vi "VI Tree.vi"   [LabVIEW 2020, in "Rohde&Schwarz CMWXP NR FR1 Measurement.lvlib"]
doc: "This is the instrument driver for the Rohde&Schwarz CMWXP NR FR1 Measurement. \n\nThe VI Tree displays all the user-callable VIs of the instrument driver in an organized table.\n\nFor detailed driver information including modification history, refer to the <B>rscmwxpnrfr1m.chm </B>file."
uses:
  <instrlib>/Rohde&Schwarz CMWXP NR FR1 Measurement/Rohde&Schwarz CMWXP NR FR1 Measurement.lvlib
panel:
  # "rsCmwxpNrFr1M"
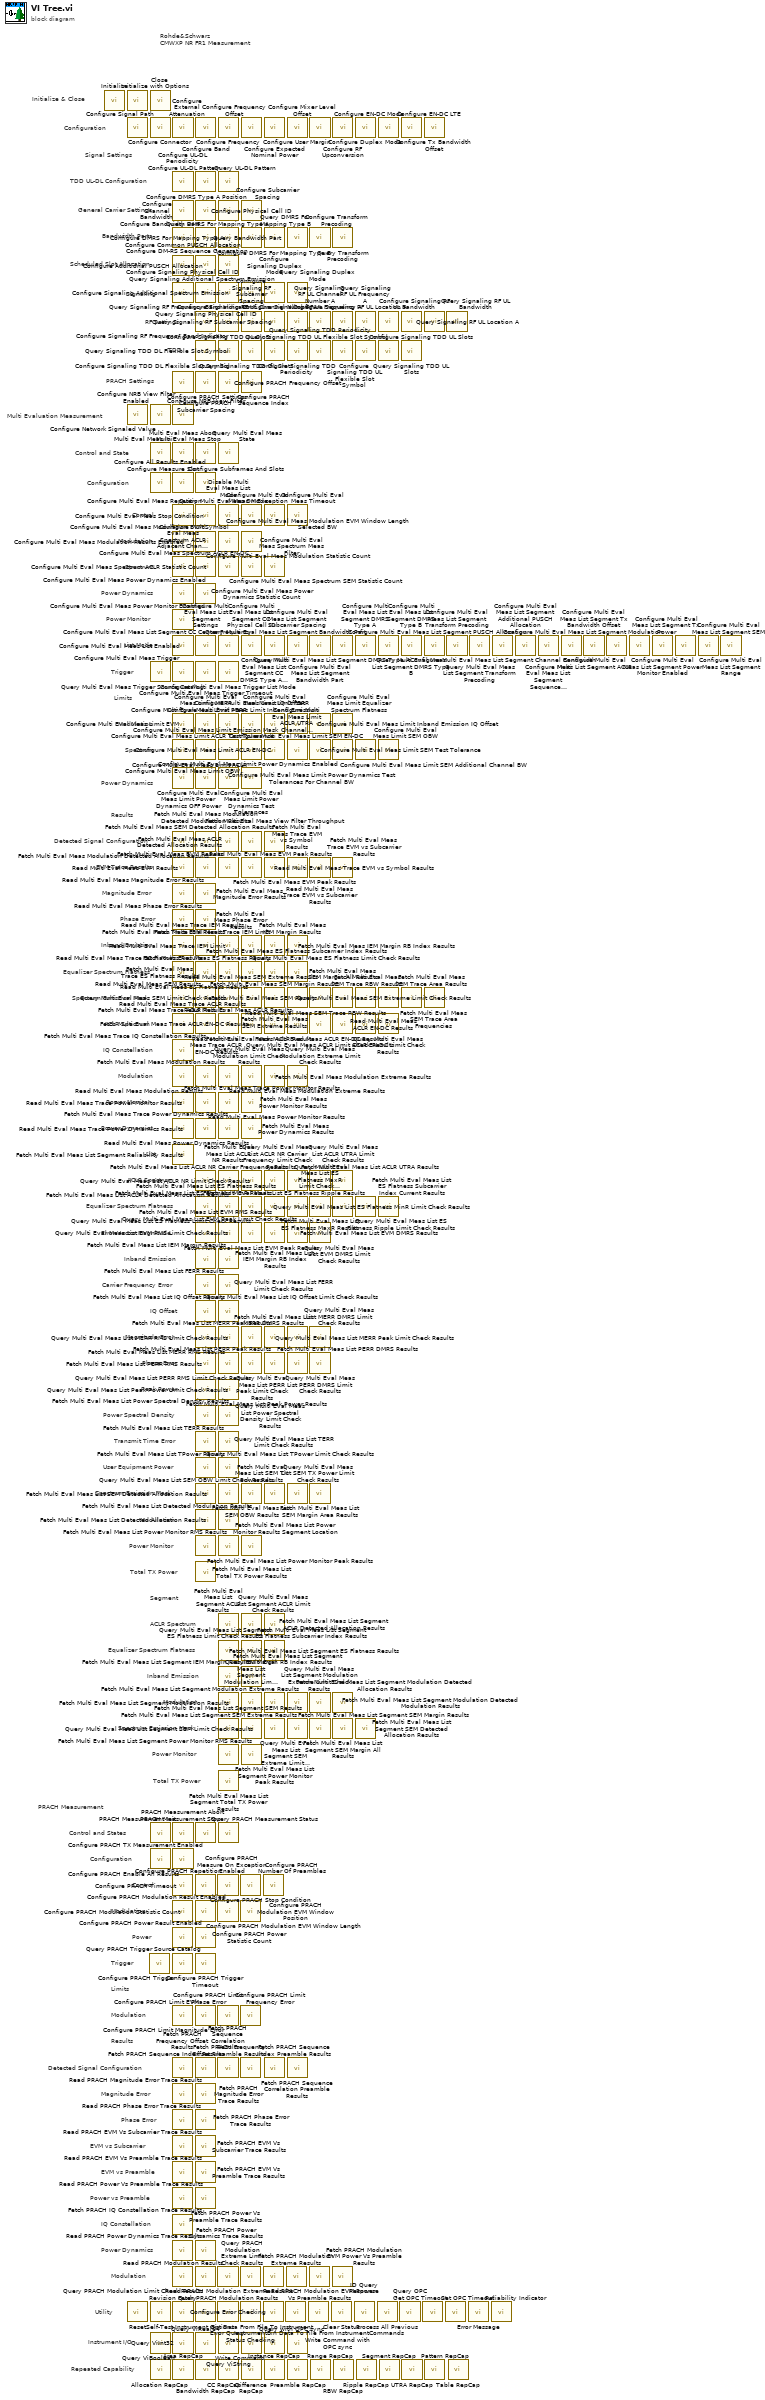
[diagram p0: block diagram]
diagram:
  # "Power Dynamics"
  # "TDD"
  # "RF Settings"
  # "Signaling"
  # "PRACH Settings"
  # "Control and State"
  # "Spectrum"
  # "Modulation"
  # "Limits"
  # "Trigger"
  # "List Mode"
  # "Power Monitor"
  # "Power Dynamics"
  # "Spectrum"
  # "Modulation"
  # "Control"
  # "Configuration"
  # "Multi Evaluation Measurement"
  # "Scheduled Slot Allocation"
  # "Bandwidth Parts"
  # "General Carrier Settings"
  # "TDD UL-DL Configuration"
  # "Signal Settings"
  # "Configuration"
  # "Total TX Power"
  # "Power Monitor"
  # "Spectrum Emission Mask"
  # "Modulation"
  # "Inband Emission"
  # "Equalizer Spectrum Flatness"
  # "ACLR Spectrum"
  # "Segment"
  # "Total TX Power"
  # "Power Monitor"
  # "Modulation"
  # "Spectrum Emission Mask"
  # "User Equipment Power"
  # "Transmit Time Error"
  # "Power Spectral Density"
  # "Peak Power"
  # "Phase Error"
  # "Magnitude Error"
  # "IQ Offset"
  # "Carrier Frequency Error"
  # "Inband Emission"
  # "Error Vector Magnitude"
  # "Equalizer Spectrum Flatness"
  # "ACLR Spectrum"
  # "List"
  # "Power Dynamics"
  # "Power Monitor"
  # "Modulation"
  # "IQ Constellation"
  # "ACLR Spectrum"
  # "Spectrum Emission Mask"
  # "Equalizer Spectrum Flatness"
  # "Inband Emission"
  # "Phase Error"
  # "Magnitude Error"
  # "EVM Trace Results"
  # "Detected Signal Configuration"
  # "Results"
  # "Modulation"
  # "Power Dynamics"
  # "IQ Constellation"
  # "Power vs Preamble"
  # "EVM vs Preamble"
  # "EVM vs Subcarrier"
  # "Phase Error"
  # "Magnitude Error"
  # "Detected Signal Configuration"
  # "Results"
  # "Modulation"
  # "Limits"
  # "Trigger"
  # "Power"
  # "Modulation"
  # "Control"
  # "Configuration"
  # "Control and States"
  # "PRACH Measurement"
  # "Repeated Capability"
  # "Rohde&Schwarz \nCMWXP NR FR1 Measurement"
  # "Instrument I/O"
  # "Utility"
  # "Initialize & Close"
  n1 = call <instrlib>:"Initialize.vi"() -> ()  [unwired: 10 in, 2 out]
  n2 = call <instrlib>:"Initialize with Options.vi"() -> ()  [unwired: 10 in, 2 out]
  n3 = call <instrlib>:"Configure Signal Path.vi"() -> ()  [unwired: 10 in, 2 out]
  n4 = call <instrlib>:"Configure Network Signaled Value.vi"() -> ()  [unwired: 10 in, 2 out]
  n5 = call <instrlib>:"Reset.vi"() -> ()  [unwired: 10 in, 2 out]
  n6 = call <instrlib>:"Configure PRACH Trigger.vi"() -> ()  [unwired: 10 in, 2 out]
  n7 = call <instrlib>:"Close.vi"() -> ()  [unwired: 11 in, 1 out]
  n8 = call <instrlib>:"Configure Connector.vi"() -> ()  [unwired: 10 in, 2 out]
  n9 = call <instrlib>:"Configure NRB View Filter Enabled.vi"() -> ()  [unwired: 10 in, 2 out]
  n10 = call <instrlib>:"Multi Eval Meas Init.vi"() -> ()  [unwired: 10 in, 2 out]
  n11 = call <instrlib>:"Configure All Results Enabled.vi"() -> ()  [unwired: 10 in, 2 out]
  n12 = call <instrlib>:"Configure Multi Eval Meas Trigger.vi"() -> ()  [unwired: 14 in, 2 out]
  n13 = call <instrlib>:"PRACH Measurement Init.vi"() -> ()  [unwired: 10 in, 2 out]
  n14 = call <instrlib>:"Configure PRACH Enable All Results.vi"() -> ()  [unwired: 10 in, 2 out]
  n15 = call <instrlib>:"Self-Test.vi"() -> ()  [unwired: 8 in, 4 out]
  n16 = call <instrlib>:"Query ViBoolean.vi"() -> ()  [unwired: 9 in, 3 out]
  n17 = call <instrlib>:"Allocation RepCap.vi"() -> ()  [unwired: 2 in, 2 out]
  n18 = call <instrlib>:"Configure PRACH Timeout.vi"() -> ()  [unwired: 10 in, 2 out]
  n19 = call <instrlib>:"Configure PRACH Modulation Statistic Count.vi"() -> ()  [unwired: 10 in, 2 out]
  n20 = call <instrlib>:"Configure PRACH Power Result Enabled.vi"() -> ()  [unwired: 10 in, 2 out]
  n21 = call <instrlib>:"Query PRACH Trigger Source Catalog.vi"() -> ()  [unwired: 9 in, 3 out]
  n22 = call <instrlib>:"Configure PRACH Limit EVM.vi"() -> ()  [unwired: 10 in, 2 out]
  n23 = call <instrlib>:"Fetch PRACH Frequency Offset Results.vi"() -> ()  [unwired: 8 in, 4 out]
  n24 = call <instrlib>:"Read PRACH Magnitude Error Trace Results.vi"() -> ()  [unwired: 8 in, 4 out]
  n25 = call <instrlib>:"Read PRACH Phase Error Trace Results.vi"() -> ()  [unwired: 8 in, 4 out]
  n26 = call <instrlib>:"Read PRACH EVM Vs Subcarrier Trace Results.vi"() -> ()  [unwired: 8 in, 4 out]
  n27 = call <instrlib>:"Read PRACH EVM Vs Preamble Trace Results.vi"() -> ()  [unwired: 8 in, 4 out]
  n28 = call <instrlib>:"Read PRACH Power Vs Preamble Trace Results.vi"() -> ()  [unwired: 8 in, 4 out]
  n29 = call <instrlib>:"Fetch PRACH IQ Constellation Trace Results.vi"() -> ()  [unwired: 8 in, 4 out]
  n30 = call <instrlib>:"Read PRACH Power Dynamics Trace Results.vi"() -> ()  [unwired: 8 in, 4 out]
  n31 = call <instrlib>:"Query PRACH Modulation Limit Check Results.vi"() -> ()  [unwired: 11 in, 5 out]
  n32 = call <instrlib>:"Configure External Attenuation.vi"() -> ()  [unwired: 10 in, 2 out]
  n33 = call <instrlib>:"Configure UL-DL Periodicity.vi"() -> ()  [unwired: 10 in, 2 out]
  n34 = call <instrlib>:"Configure Channel Bandwidth.vi"() -> ()  [unwired: 10 in, 2 out]
  n35 = call <instrlib>:"Configure Bandwidth Part.vi"() -> ()  [unwired: 14 in, 2 out]
  n36 = call <instrlib>:"Configure Common PUSCH Allocation.vi"() -> ()  [unwired: 14 in, 2 out]
  n37 = call <instrlib>:"Configure Signaling Physical Cell ID.vi"() -> ()  [unwired: 10 in, 2 out]
  n38 = call <instrlib>:"Configure PRACH Settings.vi"() -> ()  [unwired: 10 in, 2 out]
  n39 = call <instrlib>:"Configure NRB View Filter.vi"() -> ()  [unwired: 10 in, 2 out]
  n40 = call <instrlib>:"Multi Eval Meas Abort.vi"() -> ()  [unwired: 10 in, 2 out]
  n41 = call <instrlib>:"Configure Measure Slot.vi"() -> ()  [unwired: 10 in, 2 out]
  n42 = call <instrlib>:"Configure Multi Eval Meas Repetition.vi"() -> ()  [unwired: 10 in, 2 out]
  n43 = call <instrlib>:"Configure Multi Eval Meas Modulation Results Enabled.vi"() -> ()  [unwired: 10 in, 2 out]
  n44 = call <instrlib>:"Configure Multi Eval Meas Spectrum ACLR Adjacent Channel Enabled.vi"() -> ()  [unwired: 10 in, 2 out]
  n45 = call <instrlib>:"Configure Multi Eval Meas Power Dynamics Enabled.vi"() -> ()  [unwired: 10 in, 2 out]
  n46 = call <instrlib>:"Configure Multi Eval Meas Power Monitor Enabled.vi"() -> ()  [unwired: 10 in, 2 out]
  n47 = call <instrlib>:"Configure Multi Eval Meas List Enabled.vi"() -> ()  [unwired: 10 in, 2 out]
  n48 = call <instrlib>:"Query Multi Eval Meas Trigger Source Catalog.vi"() -> ()  [unwired: 9 in, 3 out]
  n49 = call <instrlib>:"Configure Multi Eval Meas Limit EVM.vi"() -> ()  [unwired: 10 in, 2 out]
  n50 = call <instrlib>:"Configure Multi Eval Meas Limit OBW.vi"() -> ()  [unwired: 10 in, 2 out]
  n51 = call <instrlib>:"Configure Multi Eval Meas Limit Power Dynamics Enabled.vi"() -> ()  [unwired: 10 in, 2 out]
  n52 = call <instrlib>:"Fetch Multi Eval Meas Modulation Detected Allocation Results.vi"() -> ()  [unwired: 8 in, 4 out]
  n53 = call <instrlib>:"Read Multi Eval Meas EVM Results.vi"() -> ()  [unwired: 8 in, 4 out]
  n54 = call <instrlib>:"Read Multi Eval Meas Magnitude Error Results.vi"() -> ()  [unwired: 8 in, 4 out]
  n55 = call <instrlib>:"Read Multi Eval Meas Phase Error Results.vi"() -> ()  [unwired: 8 in, 4 out]
  n56 = call <instrlib>:"Read Multi Eval Meas Trace IEM Results.vi"() -> ()  [unwired: 8 in, 4 out]
  n57 = call <instrlib>:"Read Multi Eval Meas Trace ES Flatness Results.vi"() -> ()  [unwired: 8 in, 4 out]
  n58 = call <instrlib>:"Read Multi Eval Meas SEM Results.vi"() -> ()  [unwired: 7 in, 5 out]
  n59 = call <instrlib>:"Read Multi Eval Meas Trace ACLR Results.vi"() -> ()  [unwired: 8 in, 4 out]
  n60 = call <instrlib>:"Fetch Multi Eval Meas Trace IQ Constellation Results.vi"() -> ()  [unwired: 8 in, 4 out]
  n61 = call <instrlib>:"Read Multi Eval Meas Modulation Results.vi"() -> ()  [unwired: 7 in, 5 out]
  n62 = call <instrlib>:"Read Multi Eval Meas Trace Power Monitor Results.vi"() -> ()  [unwired: 8 in, 4 out]
  n63 = call <instrlib>:"Read Multi Eval Meas Trace Power Dynamics Results.vi"() -> ()  [unwired: 8 in, 4 out]
  n64 = call <instrlib>:"Fetch Multi Eval Meas List Segment Reliability Results.vi"() -> ()  [unwired: 8 in, 4 out]
  n65 = call <instrlib>:"PRACH Measurement Abort.vi"() -> ()  [unwired: 10 in, 2 out]
  n66 = call <instrlib>:"Configure PRACH TX Measurement Enabled.vi"() -> ()  [unwired: 10 in, 2 out]
  n67 = call <instrlib>:"Revision Query.vi"() -> ()  [unwired: 7 in, 5 out]
  n68 = call <instrlib>:"Query ViInt32.vi"() -> ()  [unwired: 9 in, 3 out]
  n69 = call <instrlib>:"Area RepCap.vi"() -> ()  [unwired: 2 in, 2 out]
  n70 = call <instrlib>:"Configure PRACH Repetition.vi"() -> ()  [unwired: 10 in, 2 out]
  n71 = call <instrlib>:"Configure PRACH Modulation Result Enabled.vi"() -> ()  [unwired: 10 in, 2 out]
  n72 = call <instrlib>:"Configure PRACH Power Statistic Count.vi"() -> ()  [unwired: 10 in, 2 out]
  n73 = call <instrlib>:"Configure PRACH Trigger Timeout.vi"() -> ()  [unwired: 10 in, 2 out]
  n74 = call <instrlib>:"Configure PRACH Limit Magnitude Error.vi"() -> ()  [unwired: 10 in, 2 out]
  n75 = call <instrlib>:"Fetch PRACH Sequence Index Results.vi"() -> ()  [unwired: 8 in, 4 out]
  n76 = call <instrlib>:"Fetch PRACH Magnitude Error Trace Results.vi"() -> ()  [unwired: 8 in, 4 out]
  n77 = call <instrlib>:"Fetch PRACH Phase Error Trace Results.vi"() -> ()  [unwired: 8 in, 4 out]
  n78 = call <instrlib>:"Fetch PRACH EVM Vs Subcarrier Trace Results.vi"() -> ()  [unwired: 8 in, 4 out]
  n79 = call <instrlib>:"Fetch PRACH EVM Vs Preamble Trace Results.vi"() -> ()  [unwired: 8 in, 4 out]
  n80 = call <instrlib>:"Fetch PRACH Power Vs Preamble Trace Results.vi"() -> ()  [unwired: 8 in, 4 out]
  n81 = call <instrlib>:"Fetch PRACH Power Dynamics Trace Results.vi"() -> ()  [unwired: 8 in, 4 out]
  n82 = call <instrlib>:"Read PRACH Modulation Results.vi"() -> ()  [unwired: 11 in, 5 out]
  n83 = call <instrlib>:"Instrument Options.vi"() -> ()  [unwired: 9 in, 3 out]
  n84 = call <instrlib>:"Configure Band.vi"() -> ()  [unwired: 10 in, 2 out]
  n85 = call <instrlib>:"Configure UL-DL Pattern.vi"() -> ()  [unwired: 10 in, 2 out]
  n86 = call <instrlib>:"Configure Physical Cell ID.vi"() -> ()  [unwired: 10 in, 2 out]
  n87 = call <instrlib>:"Query Bandwidth Part.vi"() -> ()  [unwired: 10 in, 6 out]
  n88 = call <instrlib>:"Configure Additional PUSCH Allocation.vi"() -> ()  [unwired: 10 in, 2 out]
  n89 = call <instrlib>:"Query Signaling Physical Cell ID.vi"() -> ()  [unwired: 9 in, 3 out]
  n90 = call <instrlib>:"Configure Signaling RF Frequency Band Indicator.vi"() -> ()  [unwired: 10 in, 2 out]
  n91 = call <instrlib>:"Configure Signaling TDD DL Flexible Slot Symbol.vi"() -> ()  [unwired: 10 in, 2 out]
  n92 = call <instrlib>:"Configure PRACH Subcarrier Spacing.vi"() -> ()  [unwired: 10 in, 2 out]
  n93 = call <instrlib>:"Multi Eval Meas Stop.vi"() -> ()  [unwired: 10 in, 2 out]
  n94 = call <instrlib>:"Configure Subframes And Slots.vi"() -> ()  [unwired: 10 in, 2 out]
  n95 = call <instrlib>:"Configure Multi Eval Meas Stop Condition.vi"() -> ()  [unwired: 10 in, 2 out]
  n96 = call <instrlib>:"Configure Multi Eval Meas Modulation EVM Symbol.vi"() -> ()  [unwired: 10 in, 2 out]
  n97 = call <instrlib>:"Configure Multi Eval Meas Spectrum ACLR Statistic Count.vi"() -> ()  [unwired: 10 in, 2 out]
  n98 = call <instrlib>:"Configure Multi Eval Meas Power Dynamics Statistic Count.vi"() -> ()  [unwired: 10 in, 2 out]
  n99 = call <instrlib>:"Configure Multi Eval Meas List Segment Settings.vi"() -> ()  [unwired: 14 in, 2 out]
  n100 = call <instrlib>:"Configure Multi Eval Meas Trigger Timeout.vi"() -> ()  [unwired: 10 in, 2 out]
  n101 = call <instrlib>:"Configure Multi Eval Meas Limit MERR.vi"() -> ()  [unwired: 10 in, 2 out]
  n102 = call <instrlib>:"Configure Multi Eval Meas Limit Emission Mask.vi"() -> ()  [unwired: 14 in, 2 out]
  n103 = call <instrlib>:"Configure Multi Eval Meas Limit Power Dynamics OFF Power.vi"() -> ()  [unwired: 10 in, 2 out]
  n104 = call <instrlib>:"Fetch Multi Eval Meas Modulation Detected Modulation Results.vi"() -> ()  [unwired: 8 in, 4 out]
  n105 = call <instrlib>:"Fetch Multi Eval Meas EVM Results.vi"() -> ()  [unwired: 8 in, 4 out]
  n106 = call <instrlib>:"Fetch Multi Eval Meas Magnitude Error Results.vi"() -> ()  [unwired: 8 in, 4 out]
  n107 = call <instrlib>:"Fetch Multi Eval Meas Phase Error Results.vi"() -> ()  [unwired: 8 in, 4 out]
  n108 = call <instrlib>:"Fetch Multi Eval Meas Trace IEM Results.vi"() -> ()  [unwired: 8 in, 4 out]
  n109 = call <instrlib>:"Fetch Multi Eval Meas Trace ES Flatness Results.vi"() -> ()  [unwired: 8 in, 4 out]
  n110 = call <instrlib>:"Fetch Multi Eval Meas SEM Results.vi"() -> ()  [unwired: 7 in, 5 out]
  n111 = call <instrlib>:"Fetch Multi Eval Meas Trace ACLR Results.vi"() -> ()  [unwired: 8 in, 4 out]
  n112 = call <instrlib>:"Fetch Multi Eval Meas Modulation Results.vi"() -> ()  [unwired: 7 in, 5 out]
  n113 = call <instrlib>:"Fetch Multi Eval Meas Trace Power Monitor Results.vi"() -> ()  [unwired: 8 in, 4 out]
  n114 = call <instrlib>:"Fetch Multi Eval Meas Trace Power Dynamics Results.vi"() -> ()  [unwired: 8 in, 4 out]
  n115 = call <instrlib>:"Fetch Multi Eval Meas List ACLR Detected Allocation Results.vi"() -> ()  [unwired: 8 in, 4 out]
  n116 = call <instrlib>:"Fetch Multi Eval Meas List ES Flatness Results.vi"() -> ()  [unwired: 8 in, 4 out]
  n117 = call <instrlib>:"Fetch Multi Eval Meas List EVM RMS Results.vi"() -> ()  [unwired: 8 in, 4 out]
  n118 = call <instrlib>:"Fetch Multi Eval Meas List IEM Margin Results.vi"() -> ()  [unwired: 8 in, 4 out]
  n119 = call <instrlib>:"Fetch Multi Eval Meas List FERR Results.vi"() -> ()  [unwired: 8 in, 4 out]
  n120 = call <instrlib>:"Fetch Multi Eval Meas List IQ Offset Results.vi"() -> ()  [unwired: 8 in, 4 out]
  n121 = call <instrlib>:"Fetch Multi Eval Meas List MERR RMS Results.vi"() -> ()  [unwired: 8 in, 4 out]
  n122 = call <instrlib>:"Fetch Multi Eval Meas List PERR RMS Results.vi"() -> ()  [unwired: 8 in, 4 out]
  n123 = call <instrlib>:"Fetch Multi Eval Meas List Peak Power Results.vi"() -> ()  [unwired: 8 in, 4 out]
  n124 = call <instrlib>:"Fetch Multi Eval Meas List Power Spectral Density Results.vi"() -> ()  [unwired: 8 in, 4 out]
  n125 = call <instrlib>:"Fetch Multi Eval Meas List TERR Results.vi"() -> ()  [unwired: 8 in, 4 out]
  n126 = call <instrlib>:"Fetch Multi Eval Meas List TPower Results.vi"() -> ()  [unwired: 8 in, 4 out]
  n127 = call <instrlib>:"Fetch Multi Eval Meas List SEM Detected Allocation Results.vi"() -> ()  [unwired: 8 in, 4 out]
  n128 = call <instrlib>:"Fetch Multi Eval Meas List Detected Allocation Results.vi"() -> ()  [unwired: 8 in, 4 out]
  n129 = call <instrlib>:"Fetch Multi Eval Meas List Power Monitor RMS Results.vi"() -> ()  [unwired: 8 in, 4 out]
  n130 = call <instrlib>:"Fetch Multi Eval Meas List Total TX Power Results.vi"() -> ()  [unwired: 8 in, 4 out]
  n131 = call <instrlib>:"PRACH Measurement Stop.vi"() -> ()  [unwired: 10 in, 2 out]
  n132 = call <instrlib>:"Query ViReal64.vi"() -> ()  [unwired: 9 in, 3 out]
  n133 = call <instrlib>:"Bandwidth RepCap.vi"() -> ()  [unwired: 2 in, 2 out]
  n134 = call <instrlib>:"Configure PRACH Stop Condition.vi"() -> ()  [unwired: 10 in, 2 out]
  n135 = call <instrlib>:"Configure PRACH Modulation EVM Window Length.vi"() -> ()  [unwired: 10 in, 2 out]
  n136 = call <instrlib>:"Configure PRACH Limit Phase Error.vi"() -> ()  [unwired: 10 in, 2 out]
  n137 = call <instrlib>:"Fetch PRACH Sequence Correlation Results.vi"() -> ()  [unwired: 8 in, 4 out]
  n138 = call <instrlib>:"Fetch PRACH Modulation Results.vi"() -> ()  [unwired: 11 in, 5 out]
  n139 = call <instrlib>:"Error Query.vi"() -> ()  [unwired: 8 in, 4 out]
  n140 = call <instrlib>:"Configure Frequency.vi"() -> ()  [unwired: 10 in, 2 out]
  n141 = call <instrlib>:"Query UL-DL Pattern.vi"() -> ()  [unwired: 6 in, 6 out]
  n142 = call <instrlib>:"Configure DMRS Type A Position.vi"() -> ()  [unwired: 10 in, 2 out]
  n143 = call <instrlib>:"Configure DMRS For Mapping Type A.vi"() -> ()  [unwired: 10 in, 2 out]
  n144 = call <instrlib>:"Configure DM-RS Sequence Generation.vi"() -> ()  [unwired: 10 in, 2 out]
  n145 = call <instrlib>:"Configure Signaling Additional Spectrum Emission.vi"() -> ()  [unwired: 10 in, 2 out]
  n146 = call <instrlib>:"Query Signaling RF Frequency Band Indicator.vi"() -> ()  [unwired: 9 in, 3 out]
  n147 = call <instrlib>:"Query Signaling TDD DL Flexible Slot Symbol.vi"() -> ()  [unwired: 9 in, 3 out]
  n148 = call <instrlib>:"Configure PRACH Frequency Offset.vi"() -> ()  [unwired: 10 in, 2 out]
  n149 = call <instrlib>:"Query Multi Eval Meas State.vi"() -> ()  [unwired: 7 in, 5 out]
  n150 = call <instrlib>:"Disable Multi Eval Meas List Mode.vi"() -> ()  [unwired: 10 in, 2 out]
  n151 = call <instrlib>:"Configure Multi Eval Meas Modulation Statistic Count.vi"() -> ()  [unwired: 10 in, 2 out]
  n152 = call <instrlib>:"Configure Multi Eval Meas Spectrum ACLR EN-DC.vi"() -> ()  [unwired: 10 in, 2 out]
  n153 = call <instrlib>:"Configure Multi Eval Meas List Segment CC Center Frequency.vi"() -> ()  [unwired: 10 in, 2 out]
  n154 = call <instrlib>:"Configure Multi Eval Meas Trigger List Mode.vi"() -> ()  [unwired: 10 in, 2 out]
  n155 = call <instrlib>:"Configure Multi Eval Meas Limit PERR.vi"() -> ()  [unwired: 10 in, 2 out]
  n156 = call <instrlib>:"Configure Multi Eval Meas Limit ACLR.vi"() -> ()  [unwired: 10 in, 2 out]
  n157 = call <instrlib>:"Configure Multi Eval Meas Limit Power Dynamics Test Tolerances For Channel BW.vi"() -> ()  [unwired: 10 in, 2 out]
  n158 = call <instrlib>:"Fetch Multi Eval Meas ACLR Detected Allocation Results.vi"() -> ()  [unwired: 8 in, 4 out]
  n159 = call <instrlib>:"Read Multi Eval Meas EVM Peak Results.vi"() -> ()  [unwired: 8 in, 4 out]
  n160 = call <instrlib>:"Read Multi Eval Meas Trace IEM Limit.vi"() -> ()  [unwired: 8 in, 4 out]
  n161 = call <instrlib>:"Read Multi Eval Meas ES Flatness Results.vi"() -> ()  [unwired: 7 in, 5 out]
  n162 = call <instrlib>:"Query Multi Eval Meas SEM Limit Check Results.vi"() -> ()  [unwired: 7 in, 5 out]
  n163 = call <instrlib>:"Read Multi Eval Meas Trace ACLR EN-DC Results.vi"() -> ()  [unwired: 8 in, 4 out]
  n164 = call <instrlib>:"Query Multi Eval Meas Modulation Limit Check Results.vi"() -> ()  [unwired: 7 in, 5 out]
  n165 = call <instrlib>:"Read Multi Eval Meas Power Monitor Results.vi"() -> ()  [unwired: 7 in, 5 out]
  n166 = call <instrlib>:"Read Multi Eval Meas Power Dynamics Results.vi"() -> ()  [unwired: 7 in, 5 out]
  n167 = call <instrlib>:"Fetch Multi Eval Meas List ACLR NR Results.vi"() -> ()  [unwired: 8 in, 4 out]
  n168 = call <instrlib>:"Query Multi Eval Meas List ES Flatness Limit Check Results.vi"() -> ()  [unwired: 8 in, 4 out]
  n169 = call <instrlib>:"Query Multi Eval Meas List EVM RMS Limit Check Results.vi"() -> ()  [unwired: 8 in, 4 out]
  n170 = call <instrlib>:"Fetch Multi Eval Meas List IEM Margin RB Index Results.vi"() -> ()  [unwired: 8 in, 4 out]
  n171 = call <instrlib>:"Query Multi Eval Meas List FERR Limit Check Results.vi"() -> ()  [unwired: 8 in, 4 out]
  n172 = call <instrlib>:"Query Multi Eval Meas List IQ Offset Limit Check Results.vi"() -> ()  [unwired: 8 in, 4 out]
  n173 = call <instrlib>:"Query Multi Eval Meas List MERR RMS Limit Check Results.vi"() -> ()  [unwired: 8 in, 4 out]
  n174 = call <instrlib>:"Query Multi Eval Meas List PERR RMS Limit Check Results.vi"() -> ()  [unwired: 8 in, 4 out]
  n175 = call <instrlib>:"Query Multi Eval Meas List Peak Power Limit Check Results.vi"() -> ()  [unwired: 8 in, 4 out]
  n176 = call <instrlib>:"Query Multi Eval Meas List Power Spectral Density Limit Check Results.vi"() -> ()  [unwired: 8 in, 4 out]
  n177 = call <instrlib>:"Query Multi Eval Meas List TERR Limit Check Results.vi"() -> ()  [unwired: 8 in, 4 out]
  n178 = call <instrlib>:"Query Multi Eval Meas List TPower Limit Check Results.vi"() -> ()  [unwired: 8 in, 4 out]
  n179 = call <instrlib>:"Fetch Multi Eval Meas List SEM OBW Results.vi"() -> ()  [unwired: 8 in, 4 out]
  n180 = call <instrlib>:"Fetch Multi Eval Meas List Detected Modulation Results.vi"() -> ()  [unwired: 8 in, 4 out]
  n181 = call <instrlib>:"Fetch Multi Eval Meas List Power Monitor Peak Results.vi"() -> ()  [unwired: 8 in, 4 out]
  n182 = call <instrlib>:"Fetch Multi Eval Meas List Segment ACLR Results.vi"() -> ()  [unwired: 6 in, 6 out]
  n183 = call <instrlib>:"Fetch Multi Eval Meas List Segment ES Flatness Results.vi"() -> ()  [unwired: 6 in, 6 out]
  n184 = call <instrlib>:"Fetch Multi Eval Meas List Segment IEM Margin Results.vi"() -> ()  [unwired: 6 in, 6 out]
  n185 = call <instrlib>:"Fetch Multi Eval Meas List Segment Modulation Results.vi"() -> ()  [unwired: 6 in, 6 out]
  n186 = call <instrlib>:"Fetch Multi Eval Meas List Segment SEM Results.vi"() -> ()  [unwired: 6 in, 6 out]
  n187 = call <instrlib>:"Fetch Multi Eval Meas List Segment Power Monitor RMS Results.vi"() -> ()  [unwired: 8 in, 4 out]
  n188 = call <instrlib>:"Fetch Multi Eval Meas List Segment Total TX Power Results.vi"() -> ()  [unwired: 6 in, 6 out]
  n189 = call <instrlib>:"Query PRACH Measurement Status.vi"() -> ()  [unwired: 7 in, 5 out]
  n190 = call <instrlib>:"Query ViString.vi"() -> ()  [unwired: 9 in, 3 out]
  n191 = call <instrlib>:"CC RepCap.vi"() -> ()  [unwired: 2 in, 2 out]
  n192 = call <instrlib>:"Configure PRACH Measure On Exception Enabled.vi"() -> ()  [unwired: 10 in, 2 out]
  n193 = call <instrlib>:"Configure PRACH Modulation EVM Window Position.vi"() -> ()  [unwired: 10 in, 2 out]
  n194 = call <instrlib>:"Configure PRACH Limit Frequency Error.vi"() -> ()  [unwired: 10 in, 2 out]
  n195 = call <instrlib>:"Fetch PRACH Frequency Offset Preamble Results.vi"() -> ()  [unwired: 8 in, 4 out]
  n196 = call <instrlib>:"Query PRACH Modulation Extreme Limit Check Results.vi"() -> ()  [unwired: 7 in, 5 out]
  n197 = call <instrlib>:"Instrument Status Checking.vi"() -> ()  [unwired: 10 in, 2 out]
  n198 = call <instrlib>:"Configure Frequency Offset.vi"() -> ()  [unwired: 10 in, 2 out]
  n199 = call <instrlib>:"Configure Subcarrier Spacing.vi"() -> ()  [unwired: 10 in, 2 out]
  n200 = call <instrlib>:"Query DMRS For Mapping Type A.vi"() -> ()  [unwired: 7 in, 5 out]
  n201 = call <instrlib>:"Query Signaling Additional Spectrum Emission.vi"() -> ()  [unwired: 9 in, 3 out]
  n202 = call <instrlib>:"Configure Signaling RF Subcarrier Spacing.vi"() -> ()  [unwired: 10 in, 2 out]
  n203 = call <instrlib>:"Configure Signaling TDD DL Slots.vi"() -> ()  [unwired: 10 in, 2 out]
  n204 = call <instrlib>:"Configure PRACH Sequence Index.vi"() -> ()  [unwired: 10 in, 2 out]
  n205 = call <instrlib>:"Query Multi Eval Meas Mode.vi"() -> ()  [unwired: 9 in, 3 out]
  n206 = call <instrlib>:"Configure Multi Eval Meas Modulation EVM Window Length Selected BW.vi"() -> ()  [unwired: 10 in, 2 out]
  n207 = call <instrlib>:"Configure Multi Eval Meas Spectrum SEM Statistic Count.vi"() -> ()  [unwired: 10 in, 2 out]
  n208 = call <instrlib>:"Configure Multi Eval Meas List Segment CC Physical Cell ID.vi"() -> ()  [unwired: 10 in, 2 out]
  n209 = call <instrlib>:"Configure Multi Eval Meas Limit FERR.vi"() -> ()  [unwired: 10 in, 2 out]
  n210 = call <instrlib>:"Configure Multi Eval Meas Limit ACLR Test Tolerance.vi"() -> ()  [unwired: 10 in, 2 out]
  n211 = call <instrlib>:"Configure Multi Eval Meas Limit Power Dynamics Test Tolerances.vi"() -> ()  [unwired: 10 in, 2 out]
  n212 = call <instrlib>:"Fetch Multi Eval Meas SEM Detected Allocation Results.vi"() -> ()  [unwired: 8 in, 4 out]
  n213 = call <instrlib>:"Fetch Multi Eval Meas EVM Peak Results.vi"() -> ()  [unwired: 8 in, 4 out]
  n214 = call <instrlib>:"Fetch Multi Eval Meas Trace IEM Limit.vi"() -> ()  [unwired: 8 in, 4 out]
  n215 = call <instrlib>:"Fetch Multi Eval Meas ES Flatness Results.vi"() -> ()  [unwired: 7 in, 5 out]
  n216 = call <instrlib>:"Read Multi Eval Meas SEM Extreme Results.vi"() -> ()  [unwired: 7 in, 5 out]
  n217 = call <instrlib>:"Fetch Multi Eval Meas Trace ACLR EN-DC Results.vi"() -> ()  [unwired: 8 in, 4 out]
  n218 = call <instrlib>:"Read Multi Eval Meas Modulation Extreme Results.vi"() -> ()  [unwired: 7 in, 5 out]
  n219 = call <instrlib>:"Fetch Multi Eval Meas Power Monitor Results.vi"() -> ()  [unwired: 7 in, 5 out]
  n220 = call <instrlib>:"Fetch Multi Eval Meas Power Dynamics Results.vi"() -> ()  [unwired: 7 in, 5 out]
  n221 = call <instrlib>:"Query Multi Eval Meas List ACLR NR Limit Check Results.vi"() -> ()  [unwired: 8 in, 4 out]
  n222 = call <instrlib>:"Fetch Multi Eval Meas List ES Flatness MinR Results.vi"() -> ()  [unwired: 8 in, 4 out]
  n223 = call <instrlib>:"Fetch Multi Eval Meas List EVM Peak Results.vi"() -> ()  [unwired: 8 in, 4 out]
  n224 = call <instrlib>:"Fetch Multi Eval Meas List MERR Peak Results.vi"() -> ()  [unwired: 8 in, 4 out]
  n225 = call <instrlib>:"Fetch Multi Eval Meas List PERR Peak Results.vi"() -> ()  [unwired: 8 in, 4 out]
  n226 = call <instrlib>:"Query Multi Eval Meas List SEM OBW Limit Check Results.vi"() -> ()  [unwired: 8 in, 4 out]
  n227 = call <instrlib>:"Fetch Multi Eval Meas List Power Monitor Results Segment Location.vi"() -> ()  [unwired: 7 in, 5 out]
  n228 = call <instrlib>:"Query Multi Eval Meas List Segment ACLR Limit Check Results.vi"() -> ()  [unwired: 6 in, 6 out]
  n229 = call <instrlib>:"Query Multi Eval Meas List Segment ES Flatness Limit Check Results.vi"() -> ()  [unwired: 6 in, 6 out]
  n230 = call <instrlib>:"Fetch Multi Eval Meas List Segment IEM Margin RB Index Results.vi"() -> ()  [unwired: 6 in, 6 out]
  n231 = call <instrlib>:"Query Multi Eval Meas List Segment Modulation Limit Check Results.vi"() -> ()  [unwired: 6 in, 6 out]
  n232 = call <instrlib>:"Query Multi Eval Meas List Segment SEM Limit Check Results.vi"() -> ()  [unwired: 6 in, 6 out]
  n233 = call <instrlib>:"Fetch Multi Eval Meas List Segment Power Monitor Peak Results.vi"() -> ()  [unwired: 8 in, 4 out]
  n234 = call <instrlib>:"Write Command.vi"() -> ()  [unwired: 10 in, 2 out]
  n235 = call <instrlib>:"Difference RepCap.vi"() -> ()  [unwired: 2 in, 2 out]
  n236 = call <instrlib>:"Configure PRACH Number Of Preambles.vi"() -> ()  [unwired: 10 in, 2 out]
  n237 = call <instrlib>:"Read PRACH Modulation Extreme Results.vi"() -> ()  [unwired: 7 in, 5 out]
  n238 = call <instrlib>:"Configure Error Checking.vi"() -> ()  [unwired: 10 in, 2 out]
  n239 = call <instrlib>:"Configure Expected Nominal Power.vi"() -> ()  [unwired: 10 in, 2 out]
  n240 = call <instrlib>:"Configure DMRS For Mapping Type B.vi"() -> ()  [unwired: 10 in, 2 out]
  n241 = call <instrlib>:"Configure Signaling Duplex Mode.vi"() -> ()  [unwired: 10 in, 2 out]
  n242 = call <instrlib>:"Query Signaling RF Subcarrier Spacing.vi"() -> ()  [unwired: 9 in, 3 out]
  n243 = call <instrlib>:"Query Signaling TDD DL Slots.vi"() -> ()  [unwired: 9 in, 3 out]
  n244 = call <instrlib>:"Configure Multi Eval Meas On Exception.vi"() -> ()  [unwired: 10 in, 2 out]
  n245 = call <instrlib>:"Configure Multi Eval Meas Spectrum Meas Filter.vi"() -> ()  [unwired: 10 in, 2 out]
  n246 = call <instrlib>:"Configure Multi Eval Meas List Segment CC DMRS Type A Position.vi"() -> ()  [unwired: 10 in, 2 out]
  n247 = call <instrlib>:"Configure Multi Eval Meas Limit IQ Offset.vi"() -> ()  [unwired: 14 in, 2 out]
  n248 = call <instrlib>:"Configure Multi Eval Meas Limit ACLR EN-DC.vi"() -> ()  [unwired: 10 in, 2 out]
  n249 = call <instrlib>:"Fetch Multi Eval Meas View Filter Throughput.vi"() -> ()  [unwired: 8 in, 4 out]
  n250 = call <instrlib>:"Read Multi Eval Meas Trace EVM vs Symbol Results.vi"() -> ()  [unwired: 8 in, 4 out]
  n251 = call <instrlib>:"Fetch Multi Eval Meas IEM Margin Results.vi"() -> ()  [unwired: 7 in, 5 out]
  n252 = call <instrlib>:"Query Multi Eval Meas ES Flatness Limit Check Results.vi"() -> ()  [unwired: 7 in, 5 out]
  n253 = call <instrlib>:"Fetch Multi Eval Meas SEM Extreme Results.vi"() -> ()  [unwired: 7 in, 5 out]
  n254 = call <instrlib>:"Read Multi Eval Meas ACLR Results.vi"() -> ()  [unwired: 8 in, 4 out]
  n255 = call <instrlib>:"Fetch Multi Eval Meas Modulation Extreme Results.vi"() -> ()  [unwired: 7 in, 5 out]
  n256 = call <instrlib>:"Fetch Multi Eval Meas List ACLR NR Carrier Frequency Results.vi"() -> ()  [unwired: 8 in, 4 out]
  n257 = call <instrlib>:"Query Multi Eval Meas List ES Flatness MinR Limit Check Results.vi"() -> ()  [unwired: 8 in, 4 out]
  n258 = call <instrlib>:"Query Multi Eval Meas List EVM Peak Limit Check Results.vi"() -> ()  [unwired: 8 in, 4 out]
  n259 = call <instrlib>:"Query Multi Eval Meas List MERR Peak Limit Check Results.vi"() -> ()  [unwired: 8 in, 4 out]
  n260 = call <instrlib>:"Query Multi Eval Meas List PERR Peak Limit Check Results.vi"() -> ()  [unwired: 8 in, 4 out]
  n261 = call <instrlib>:"Fetch Multi Eval Meas List SEM TX Power Results.vi"() -> ()  [unwired: 8 in, 4 out]
  n262 = call <instrlib>:"Fetch Multi Eval Meas List Segment ACLR Detected Allocation Results.vi"() -> ()  [unwired: 8 in, 4 out]
  n263 = call <instrlib>:"Fetch Multi Eval Meas List Segment ES Flatness Subcarrier Index Results.vi"() -> ()  [unwired: 6 in, 6 out]
  n264 = call <instrlib>:"Fetch Multi Eval Meas List Segment Modulation Extreme Results.vi"() -> ()  [unwired: 6 in, 6 out]
  n265 = call <instrlib>:"Fetch Multi Eval Meas List Segment SEM Extreme Results.vi"() -> ()  [unwired: 6 in, 6 out]
  n266 = call <instrlib>:"Fetch PRACH Sequence Index Preamble Results.vi"() -> ()  [unwired: 8 in, 4 out]
  n267 = call <instrlib>:"Query with OPC sync.vi"() -> ()  [unwired: 9 in, 3 out]
  n268 = call <instrlib>:"Instance RepCap.vi"() -> ()  [unwired: 2 in, 2 out]
  n269 = call <instrlib>:"Bin Data From File To Instrument.vi"() -> ()  [unwired: 10 in, 2 out]
  n270 = call <instrlib>:"Fetch PRACH Modulation Extreme Results.vi"() -> ()  [unwired: 7 in, 5 out]
  n271 = call <instrlib>:"Configure User Margin.vi"() -> ()  [unwired: 10 in, 2 out]
  n272 = call <instrlib>:"Query DMRS For Mapping Type B.vi"() -> ()  [unwired: 7 in, 5 out]
  n273 = call <instrlib>:"Query Signaling Duplex Mode.vi"() -> ()  [unwired: 9 in, 3 out]
  n274 = call <instrlib>:"Configure Signaling RF UL Channel Number A.vi"() -> ()  [unwired: 10 in, 2 out]
  n275 = call <instrlib>:"Configure Signaling TDD Periodicity.vi"() -> ()  [unwired: 10 in, 2 out]
  n276 = call <instrlib>:"Configure Multi Eval Meas Timeout.vi"() -> ()  [unwired: 10 in, 2 out]
  n277 = call <instrlib>:"Configure Multi Eval Meas List Segment Subcarrier Spacing.vi"() -> ()  [unwired: 10 in, 2 out]
  n278 = call <instrlib>:"Configure Multi Eval Meas Limit Inband Emission.vi"() -> ()  [unwired: 14 in, 2 out]
  n279 = call <instrlib>:"Configure Multi Eval Meas Limit ACLR UTRA Channel Bandwidth.vi"() -> ()  [unwired: 14 in, 2 out]
  n280 = call <instrlib>:"Fetch Multi Eval Meas Trace EVM vs Symbol Results.vi"() -> ()  [unwired: 8 in, 4 out]
  n281 = call <instrlib>:"Fetch Multi Eval Meas IEM Margin RB Index Results.vi"() -> ()  [unwired: 12 in, 4 out]
  n282 = call <instrlib>:"Fetch Multi Eval Meas ES Flatness Subcarrier Index Results.vi"() -> ()  [unwired: 7 in, 5 out]
  n283 = call <instrlib>:"Query Multi Eval Meas SEM Extreme Limit Check Results.vi"() -> ()  [unwired: 7 in, 5 out]
  n284 = call <instrlib>:"Fetch Multi Eval Meas ACLR Results.vi"() -> ()  [unwired: 8 in, 4 out]
  n285 = call <instrlib>:"Query Multi Eval Meas Modulation Extreme Limit Check Results.vi"() -> ()  [unwired: 7 in, 5 out]
  n286 = call <instrlib>:"Query Multi Eval Meas List ACLR NR Carrier Frequency Limit Check Results.vi"() -> ()  [unwired: 8 in, 4 out]
  n287 = call <instrlib>:"Fetch Multi Eval Meas List ES Flatness MaxR Results.vi"() -> ()  [unwired: 8 in, 4 out]
  n288 = call <instrlib>:"Fetch Multi Eval Meas List EVM DMRS Results.vi"() -> ()  [unwired: 8 in, 4 out]
  n289 = call <instrlib>:"Fetch Multi Eval Meas List MERR DMRS Results.vi"() -> ()  [unwired: 8 in, 4 out]
  n290 = call <instrlib>:"Fetch Multi Eval Meas List PERR DMRS Results.vi"() -> ()  [unwired: 8 in, 4 out]
  n291 = call <instrlib>:"Query Multi Eval Meas List SEM TX Power Limit Check Results.vi"() -> ()  [unwired: 8 in, 4 out]
  n292 = call <instrlib>:"Query Multi Eval Meas List Segment Modulation Extreme Limit Check Results.vi"() -> ()  [unwired: 6 in, 6 out]
  n293 = call <instrlib>:"Query Multi Eval Meas List Segment SEM Extreme Limit Check Results.vi"() -> ()  [unwired: 6 in, 6 out]
  n294 = call <instrlib>:"Fetch PRACH Sequence Correlation Preamble Results.vi"() -> ()  [unwired: 8 in, 4 out]
  n295 = call <instrlib>:"Write Command with OPC sync.vi"() -> ()  [unwired: 10 in, 2 out]
  n296 = call <instrlib>:"Preamble RepCap.vi"() -> ()  [unwired: 2 in, 2 out]
  n297 = call <instrlib>:"Bin Data To File From Instrument.vi"() -> ()  [unwired: 10 in, 2 out]
  n298 = call <instrlib>:"Read PRACH Modulation EVM Power Vs Preamble Results.vi"() -> ()  [unwired: 11 in, 5 out]
  n299 = call <instrlib>:"Configure Mixer Level Offset.vi"() -> ()  [unwired: 10 in, 2 out]
  n300 = call <instrlib>:"Configure Transform Precoding.vi"() -> ()  [unwired: 10 in, 2 out]
  n301 = call <instrlib>:"Query Signaling RF UL Channel Number A.vi"() -> ()  [unwired: 9 in, 3 out]
  n302 = call <instrlib>:"Query Signaling TDD Periodicity.vi"() -> ()  [unwired: 9 in, 3 out]
  n303 = call <instrlib>:"Configure Multi Eval Meas List Segment Bandwidth Part.vi"() -> ()  [unwired: 14 in, 2 out]
  n304 = call <instrlib>:"Configure Multi Eval Meas Limit Inband Emission IQ Offset.vi"() -> ()  [unwired: 10 in, 2 out]
  n305 = call <instrlib>:"Configure Multi Eval Meas Limit SEM Test Tolerance.vi"() -> ()  [unwired: 10 in, 2 out]
  n306 = call <instrlib>:"Read Multi Eval Meas Trace EVM vs Subcarrier Results.vi"() -> ()  [unwired: 8 in, 4 out]
  n307 = call <instrlib>:"Fetch Multi Eval Meas SEM Margin Results.vi"() -> ()  [unwired: 7 in, 5 out]
  n308 = call <instrlib>:"Query Multi Eval Meas ACLR Limit Check Results.vi"() -> ()  [unwired: 8 in, 4 out]
  n309 = call <instrlib>:"Fetch Multi Eval Meas List ACLR UTRA Results.vi"() -> ()  [unwired: 8 in, 4 out]
  n310 = call <instrlib>:"Query Multi Eval Meas List ES Flatness MaxR Limit Check Results.vi"() -> ()  [unwired: 8 in, 4 out]
  n311 = call <instrlib>:"Query Multi Eval Meas List EVM DMRS Limit Check Results.vi"() -> ()  [unwired: 8 in, 4 out]
  n312 = call <instrlib>:"Query Multi Eval Meas List MERR DMRS Limit Check Results.vi"() -> ()  [unwired: 8 in, 4 out]
  n313 = call <instrlib>:"Query Multi Eval Meas List PERR DMRS Limit Check Results.vi"() -> ()  [unwired: 8 in, 4 out]
  n314 = call <instrlib>:"Fetch Multi Eval Meas List SEM Margin Area Results.vi"() -> ()  [unwired: 8 in, 4 out]
  n315 = call <instrlib>:"Fetch Multi Eval Meas List Segment Modulation Detected Allocation Results.vi"() -> ()  [unwired: 8 in, 4 out]
  n316 = call <instrlib>:"Fetch Multi Eval Meas List Segment SEM Margin Results.vi"() -> ()  [unwired: 6 in, 6 out]
  n317 = call <instrlib>:"Range RepCap.vi"() -> ()  [unwired: 2 in, 2 out]
  n318 = call <instrlib>:"Clear Status.vi"() -> ()  [unwired: 10 in, 2 out]
  n319 = call <instrlib>:"Fetch PRACH Modulation EVM Power Vs Preamble Results.vi"() -> ()  [unwired: 11 in, 5 out]
  n320 = call <instrlib>:"Configure RF Upconversion.vi"() -> ()  [unwired: 10 in, 2 out]
  n321 = call <instrlib>:"Query Transform Precoding.vi"() -> ()  [unwired: 9 in, 3 out]
  n322 = call <instrlib>:"Configure Signaling RF UL Frequency A.vi"() -> ()  [unwired: 10 in, 2 out]
  n323 = call <instrlib>:"Configure Signaling TDD UL Flexible Slot Symbol.vi"() -> ()  [unwired: 10 in, 2 out]
  n324 = call <instrlib>:"Query Multi Eval Meas List Segment Bandwidth Part.vi"() -> ()  [unwired: 10 in, 6 out]
  n325 = call <instrlib>:"Configure Multi Eval Meas Limit Equalizer Spectrum Flatness.vi"() -> ()  [unwired: 14 in, 2 out]
  n326 = call <instrlib>:"Configure Multi Eval Meas Limit SEM EN-DC.vi"() -> ()  [unwired: 14 in, 2 out]
  n327 = call <instrlib>:"Fetch Multi Eval Meas Trace EVM vs Subcarrier Results.vi"() -> ()  [unwired: 8 in, 4 out]
  n328 = call <instrlib>:"Fetch Multi Eval Meas SEM Margin All Results.vi"() -> ()  [unwired: 7 in, 5 out]
  n329 = call <instrlib>:"Read Multi Eval Meas ACLR EN-DC Results.vi"() -> ()  [unwired: 8 in, 4 out]
  n330 = call <instrlib>:"Query Multi Eval Meas List ACLR UTRA Limit Check Results.vi"() -> ()  [unwired: 8 in, 4 out]
  n331 = call <instrlib>:"Fetch Multi Eval Meas List ES Flatness Ripple Results.vi"() -> ()  [unwired: 8 in, 4 out]
  n332 = call <instrlib>:"Fetch Multi Eval Meas List Segment Modulation Detected Modulation Results.vi"() -> ()  [unwired: 8 in, 4 out]
  n333 = call <instrlib>:"Fetch Multi Eval Meas List Segment SEM Margin All Results.vi"() -> ()  [unwired: 6 in, 6 out]
  n334 = call <instrlib>:"RBW RepCap.vi"() -> ()  [unwired: 2 in, 2 out]
  n335 = call <instrlib>:"ID Query Response.vi"() -> ()  [unwired: 9 in, 3 out]
  n336 = call <instrlib>:"Configure Duplex Mode.vi"() -> ()  [unwired: 10 in, 2 out]
  n337 = call <instrlib>:"Query Signaling RF UL Frequency A.vi"() -> ()  [unwired: 9 in, 3 out]
  n338 = call <instrlib>:"Query Signaling TDD UL Flexible Slot Symbol.vi"() -> ()  [unwired: 9 in, 3 out]
  n339 = call <instrlib>:"Configure Multi Eval Meas List Segment DMRS Type A.vi"() -> ()  [unwired: 14 in, 2 out]
  n340 = call <instrlib>:"Configure Multi Eval Meas Limit SEM Additional Channel BW.vi"() -> ()  [unwired: 14 in, 2 out]
  n341 = call <instrlib>:"Read Multi Eval Meas SEM Trace RBW Results.vi"() -> ()  [unwired: 8 in, 4 out]
  n342 = call <instrlib>:"Fetch Multi Eval Meas ACLR EN-DC Results.vi"() -> ()  [unwired: 8 in, 4 out]
  n343 = call <instrlib>:"Query Multi Eval Meas List ES Flatness Ripple Limit Check Results.vi"() -> ()  [unwired: 8 in, 4 out]
  n344 = call <instrlib>:"Fetch Multi Eval Meas List Segment SEM Detected Allocation Results.vi"() -> ()  [unwired: 8 in, 4 out]
  n345 = call <instrlib>:"Ripple RepCap.vi"() -> ()  [unwired: 2 in, 2 out]
  n346 = call <instrlib>:"Process All Previous Commands.vi"() -> ()  [unwired: 10 in, 2 out]
  n347 = call <instrlib>:"Configure EN-DC Mode.vi"() -> ()  [unwired: 10 in, 2 out]
  n348 = call <instrlib>:"Configure Signaling RF UL Location A.vi"() -> ()  [unwired: 10 in, 2 out]
  n349 = call <instrlib>:"Configure Signaling TDD UL Slots.vi"() -> ()  [unwired: 10 in, 2 out]
  n350 = call <instrlib>:"Query Multi Eval Meas List Segment DMRS Type A.vi"() -> ()  [unwired: 11 in, 5 out]
  n351 = call <instrlib>:"Configure Multi Eval Meas Limit SEM OBW.vi"() -> ()  [unwired: 10 in, 2 out]
  n352 = call <instrlib>:"Fetch Multi Eval Meas SEM Trace RBW Results.vi"() -> ()  [unwired: 8 in, 4 out]
  n353 = call <instrlib>:"Query Multi Eval Meas ACLR EN-DC Limit Check Results.vi"() -> ()  [unwired: 8 in, 4 out]
  n354 = call <instrlib>:"Fetch Multi Eval Meas List ES Flatness Subcarrier Index Current Results.vi"() -> ()  [unwired: 8 in, 4 out]
  n355 = call <instrlib>:"Segment RepCap.vi"() -> ()  [unwired: 2 in, 2 out]
  n356 = call <instrlib>:"Query OPC.vi"() -> ()  [unwired: 9 in, 3 out]
  n357 = call <instrlib>:"Configure EN-DC LTE.vi"() -> ()  [unwired: 10 in, 2 out]
  n358 = call <instrlib>:"Query Signaling RF UL Location A.vi"() -> ()  [unwired: 9 in, 3 out]
  n359 = call <instrlib>:"Query Signaling TDD UL Slots.vi"() -> ()  [unwired: 9 in, 3 out]
  n360 = call <instrlib>:"Configure Multi Eval Meas List Segment DMRS Type B.vi"() -> ()  [unwired: 14 in, 2 out]
  n361 = call <instrlib>:"Fetch Multi Eval Meas SEM Trace Area Results.vi"() -> ()  [unwired: 7 in, 5 out]
  n362 = call <instrlib>:"UTRA RepCap.vi"() -> ()  [unwired: 2 in, 2 out]
  n363 = call <instrlib>:"Get OPC Timeout.vi"() -> ()  [unwired: 9 in, 3 out]
  n364 = call <instrlib>:"Configure Tx Bandwidth Offset.vi"() -> ()  [unwired: 10 in, 2 out]
  n365 = call <instrlib>:"Configure Signaling RF UL Bandwidth.vi"() -> ()  [unwired: 10 in, 2 out]
  n366 = call <instrlib>:"Query Multi Eval Meas List Segment DMRS Type B.vi"() -> ()  [unwired: 11 in, 5 out]
  n367 = call <instrlib>:"Fetch Multi Eval Meas SEM Trace Area Frequencies.vi"() -> ()  [unwired: 7 in, 5 out]
  n368 = call <instrlib>:"Pattern RepCap.vi"() -> ()  [unwired: 2 in, 2 out]
  n369 = call <instrlib>:"Set OPC Timeout.vi"() -> ()  [unwired: 10 in, 2 out]
  n370 = call <instrlib>:"Query Signaling RF UL Bandwidth.vi"() -> ()  [unwired: 9 in, 3 out]
  n371 = call <instrlib>:"Configure Multi Eval Meas List Segment Transform Precoding.vi"() -> ()  [unwired: 10 in, 2 out]
  n372 = call <instrlib>:"Table RepCap.vi"() -> ()  [unwired: 2 in, 2 out]
  n373 = call <instrlib>:"Error Message.vi"() -> ()  [unwired: 7 in, 5 out]
  n374 = call <instrlib>:"Query Multi Eval Meas List Segment Transform Precoding.vi"() -> ()  [unwired: 9 in, 3 out]
  n375 = call <instrlib>:"Reliability Indicator.vi"() -> ()  [unwired: 9 in, 3 out]
  n376 = call <instrlib>:"Configure Multi Eval Meas List Segment PUSCH Allocation.vi"() -> ()  [unwired: 14 in, 2 out]
  n377 = call <instrlib>:"Configure Multi Eval Meas List Segment Additional PUSCH Allocation.vi"() -> ()  [unwired: 10 in, 2 out]
  n378 = call <instrlib>:"Configure Multi Eval Meas List Segment Sequence Generation.vi"() -> ()  [unwired: 14 in, 2 out]
  n379 = call <instrlib>:"Configure Multi Eval Meas List Segment Channel Bandwidth.vi"() -> ()  [unwired: 10 in, 2 out]
  n380 = call <instrlib>:"Configure Multi Eval Meas List Segment Tx Bandwidth Offset.vi"() -> ()  [unwired: 10 in, 2 out]
  n381 = call <instrlib>:"Configure Multi Eval Meas List Segment ACLR.vi"() -> ()  [unwired: 14 in, 2 out]
  n382 = call <instrlib>:"Configure Multi Eval Meas List Segment Modulation.vi"() -> ()  [unwired: 14 in, 2 out]
  n383 = call <instrlib>:"Configure Multi Eval Meas List Segment Power Monitor Enabled.vi"() -> ()  [unwired: 10 in, 2 out]
  n384 = call <instrlib>:"Configure Multi Eval Meas List Segment Tx Power.vi"() -> ()  [unwired: 10 in, 2 out]
  n385 = call <instrlib>:"Configure Multi Eval Meas List Segment SEM.vi"() -> ()  [unwired: 10 in, 2 out]
  n386 = call <instrlib>:"Configure Multi Eval Meas List Segment Range.vi"() -> ()  [unwired: 10 in, 2 out]
